vi "python simple example array.vi"() -> ()   [LabVIEW 2018]
panel:
  out "return value":string
  in  "Python version":string="3.8"
  in  "function name":string="callme"
  in  "module path":path=path "C:/Users/tony_/Downloads/2020_04_24_PNG_HDF5_Benchmark_Tony/2020_04_24_PNG_HDF5_Benchmark_Tony/arraytest.py"
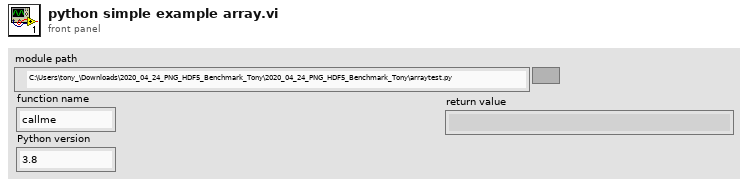
[diagram p1: front panel]
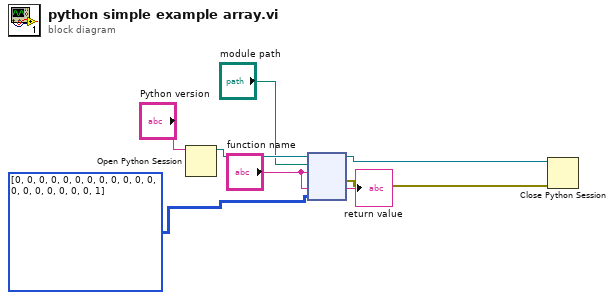
[diagram p0: block diagram]
diagram:
  n1 = Open Python Session(python version="Python version") -> (session out=w7:refnum<k35>)  [unwired: 2 in, 1 out]
  n2 = node(w7, "module path", "function name", "function name", u16[][] [[0, 0, 0, 0, 0], [0, 0, 0, 0, 0], [0, 0, 0, 0, 0], [0, 0, 0, 0, 1]]) -> (w6:refnum<k35>, w5:errorcluster, →"return value":string)  [unwired: 2 in, 2 out]
  n3 = Close Python Session(session in=w6, error in=w5) -> ()  [unwired: 1 out]
